vi "RSA Encrypt.vi"(7 "public key":string, 8 "error in (no error)":errorcluster, 10 "data":u8[](array[numeric]), 11 "RSA in":refnum<class "RSA.lvclass">) -> (0 "error out":errorcluster, 2 "encrypted_data":u8[](array[numeric]), 3 "RSA out":refnum<class "RSA.lvclass">)   [LabVIEW 2023, in "RSA.lvclass"]
uses:
  RSA.lvclass
  RSA.lvclass/RSA.ctl
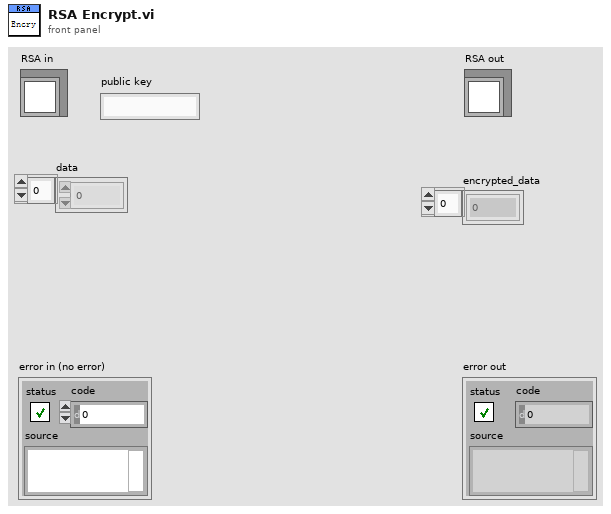
[diagram p1: front panel]
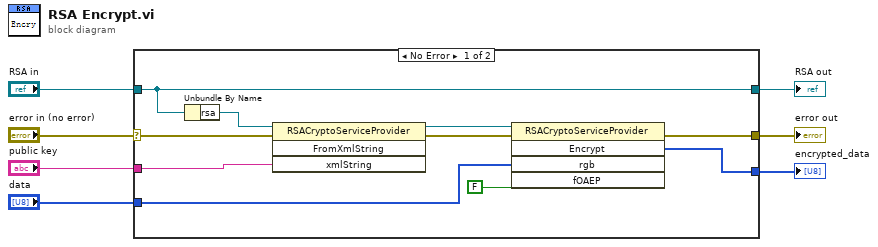
[diagram p0: block diagram]
diagram:
  n1 = case shown="No Error" "error in (no error)" {
    selector: "error in (no error)" -> [w12 w19]
    tunnel: [w9 w19] -> w6
    tunnel: [w11 w18] -> w4
    tunnel: "RSA in" -> [w11 w18]
    tunnel: "public key" -> [w17 _]
    tunnel: [w13 _] -> w2
    tunnel: "data" -> [w8 _]
    frame No Error {
      n2 = Unbundle By Name(w11) -> ("rsa"=w10:refnum<k24>)
      n3 = invoke class="RSACryptoServiceProvider" method="FromXmlString"(reference=w10, error in=w12, "xmlString"=w17) -> (reference out=w15:refnum<k24>, error out=w16:errorcluster)  [unwired: 1 in, 2 out]
      n4 = invoke class="RSACryptoServiceProvider" method="Encrypt"(reference=w15, error in=w16, "rgb"=w8, "fOAEP"=FALSE) -> (error out=w9:errorcluster, "Encrypt"=w13:u8[])  [unwired: 1 in, 3 out]
    }
    frame Error {
    }
  }
  "error out" <- w6
  "RSA out" <- w4
  "encrypted_data" <- w2
